vi "FPGA_Digital Output.vi"(10 "Digital Output Data":T1, 11 "Digital Output":T2={"DO 0"="RMC/DIO62", "DO 1"="RMC/DIO44", "DO 2"="RMC/DIO77", "DO 3"="RMC/DIO61", "DO 4"="RMC/DIO94", "DO 5"="RMC/DIO12", "DO 6"="RMC/DIO76", "DO 7"="RMC/DIO29", "DO 8"="RMC/DIO93", "DO 9"="RMC/DIO11", "DO 10"="RMC/DIO43", "DO 11"="RMC/DIO28"}) -> ()   [LabVIEW 2018]
uses:
  Data Def/FPGA_Digital Output.ctl
  Data Def/FPGA_Digital Output Data.ctl
  <vilib>/rvi/eio/common/nirviEmuTemplateMethod_errors.vi
  <vilib>/eio/EIONode/EIONode.xnode
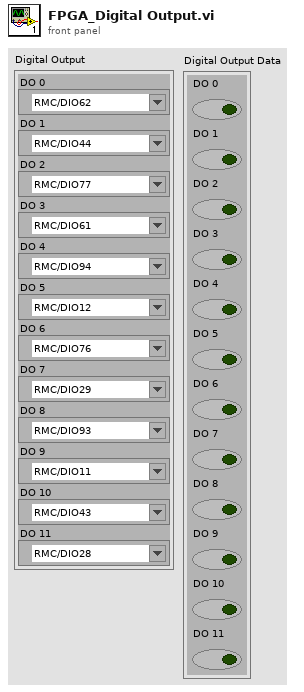
[diagram p1: front panel]
types:
  T1 = typedef "FPGA_Digital Output Data.ctl" = cluster{"DO 0":bool, "DO 1":bool, "DO 2":bool, "DO 3":bool, "DO 4":bool, "DO 5":bool, "DO 6":bool, "DO 7":bool, "DO 8":bool, "DO 9":bool, "DO 10":bool, "DO 11":bool}
  T2 = typedef "FPGA_Digital Output.ctl" = cluster{"DO 0":refnum<k21>, "DO 1":refnum<k21>, "DO 2":refnum<k21>, "DO 3":refnum<k21>, "DO 4":refnum<k21>, "DO 5":refnum<k21>, "DO 6":refnum<k21>, "DO 7":refnum<k21>, "DO 8":refnum<k21>, "DO 9":refnum<k21>, "DO 10":refnum<k21>, "DO 11":refnum<k21>}
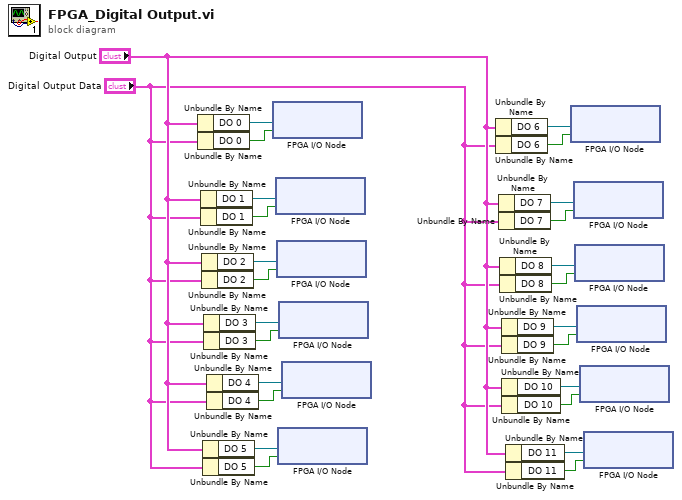
[diagram p0: block diagram]
diagram:
  n1 = Unbundle By Name("Digital Output") -> ("DO 0"=w26:refnum<k21>)
  n2 = Unbundle By Name("Digital Output Data") -> ("DO 0"=w25:bool)
  n3 = Unbundle By Name("Digital Output") -> ("DO 1"=w23:refnum<k21>)
  n4 = Unbundle By Name("Digital Output Data") -> ("DO 1"=w24:bool)
  n5 = Unbundle By Name("Digital Output") -> ("DO 2"=w22:refnum<k21>)
  n6 = Unbundle By Name("Digital Output Data") -> ("DO 2"=w21:bool)
  n7 = Unbundle By Name("Digital Output") -> ("DO 5"=w15:refnum<k21>)
  n8 = Unbundle By Name("Digital Output Data") -> ("DO 5"=w16:bool)
  n9 = Unbundle By Name("Digital Output") -> ("DO 3"=w19:refnum<k21>)
  n10 = Unbundle By Name("Digital Output Data") -> ("DO 3"=w20:bool)
  n11 = Unbundle By Name("Digital Output") -> ("DO 4"=w18:refnum<k21>)
  n12 = Unbundle By Name("Digital Output Data") -> ("DO 4"=w17:bool)
  n13 = xnode "FPGA I/O Node"("I/O Item"=w25, "FPGA I/O In"=w26) -> ()  [unwired: 1 out]
  n14 = xnode "FPGA I/O Node"("I/O Item"=w24, "FPGA I/O In"=w23) -> ()  [unwired: 1 out]
  n15 = xnode "FPGA I/O Node"("I/O Item"=w21, "FPGA I/O In"=w22) -> ()  [unwired: 1 out]
  n16 = xnode "FPGA I/O Node"("I/O Item"=w16, "FPGA I/O In"=w15) -> ()  [unwired: 1 out]
  n17 = xnode "FPGA I/O Node"("I/O Item"=w20, "FPGA I/O In"=w19) -> ()  [unwired: 1 out]
  n18 = xnode "FPGA I/O Node"("I/O Item"=w17, "FPGA I/O In"=w18) -> ()  [unwired: 1 out]
  n19 = Unbundle By Name("Digital Output") -> ("DO 6"=w3:refnum<k21>)
  n20 = Unbundle By Name("Digital Output Data") -> ("DO 6"=w4:bool)
  n21 = Unbundle By Name("Digital Output") -> ("DO 7"=w6:refnum<k21>)
  n22 = Unbundle By Name("Digital Output Data") -> ("DO 7"=w5:bool)
  n23 = Unbundle By Name("Digital Output") -> ("DO 8"=w7:refnum<k21>)
  n24 = Unbundle By Name("Digital Output Data") -> ("DO 8"=w8:bool)
  n25 = Unbundle By Name("Digital Output") -> ("DO 9"=w10:refnum<k21>)
  n26 = Unbundle By Name("Digital Output Data") -> ("DO 9"=w9:bool)
  n27 = Unbundle By Name("Digital Output") -> ("DO 10"=w11:refnum<k21>)
  n28 = Unbundle By Name("Digital Output Data") -> ("DO 10"=w12:bool)
  n29 = Unbundle By Name("Digital Output") -> ("DO 11"=w14:refnum<k21>)
  n30 = Unbundle By Name("Digital Output Data") -> ("DO 11"=w13:bool)
  n31 = xnode "FPGA I/O Node"("I/O Item"=w4, "FPGA I/O In"=w3) -> ()  [unwired: 1 out]
  n32 = xnode "FPGA I/O Node"("I/O Item"=w5, "FPGA I/O In"=w6) -> ()  [unwired: 1 out]
  n33 = xnode "FPGA I/O Node"("I/O Item"=w8, "FPGA I/O In"=w7) -> ()  [unwired: 1 out]
  n34 = xnode "FPGA I/O Node"("I/O Item"=w9, "FPGA I/O In"=w10) -> ()  [unwired: 1 out]
  n35 = xnode "FPGA I/O Node"("I/O Item"=w12, "FPGA I/O In"=w11) -> ()  [unwired: 1 out]
  n36 = xnode "FPGA I/O Node"("I/O Item"=w13, "FPGA I/O In"=w14) -> ()  [unwired: 1 out]
